vi "Handle.vi"(7 "Queue in":refnum<class "Queue.lvclass">, 11 "State in":refnum<class "State.lvclass">) -> (2 "Destroy?":bool, 5 "Queue out":refnum<class "Queue.lvclass">)   [LabVIEW 2021, in "jettl.lvlib" / "Base Queue.lvlib" / "State.lvlib" / "State.lvclass"]
uses:
  State.lvclass
  Queue/Queue.lvclass
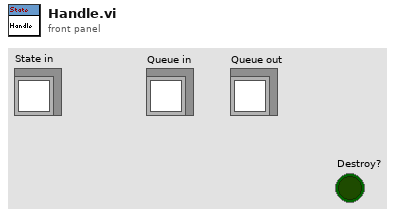
[diagram p1: front panel]
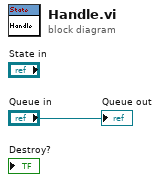
[diagram p0: block diagram]
diagram:
  "Queue out" <- "Queue in"
